vi "Disable Controls.vi"(7 "Disabled":T1(ring), 8 "error in (no error)":errorcluster, 11 "array":refnum<vi>[](array[refnum])) -> (0 "error out":errorcluster)   [LabVIEW 2013]
doc: "Use this VI to disable/enable all protocol controls."
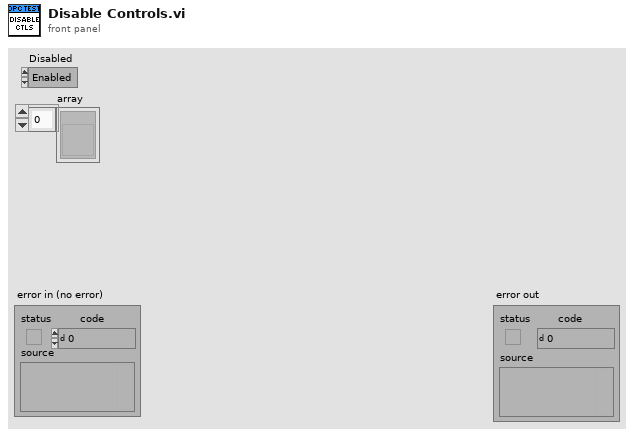
[diagram p1: front panel]
types:
  T1 = enum8{"Enabled", "Disabled", "Disabled and Grayed Out"}
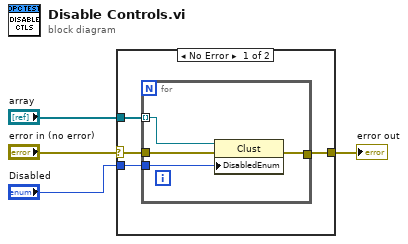
[diagram p0: block diagram]
diagram:
  n1 = case shown="No Error" "error in (no error)" {
    selector: "error in (no error)" -> [w6 w13]
    tunnel: [w5 w13] -> w3
    tunnel: "array" -> [w8 _]
    tunnel: "Disabled" -> [w7 _]
    frame No Error {
      n2 = for {
        tunnel: w8 -> [w12] mode=indexing
        tunnel: w7 -> [w11]
        tunnel: w6 -> [w10]
        tunnel: [w9] -> w5
        n3 = property class="Clust"(reference=w12, error in=w10, "DisabledEnum"=w11) -> (error out=w9:errorcluster)  [unwired: 1 out]
      }
    }
    frame Error {
    }
  }
  "error out" <- w3
